vi "T257P_Check_Temperature.vi"(0 "T257P Port IN":refnum<visa-resource-name>, 5 "error in (no error)":errorcluster) -> (7 "Sent buffer 1":string, 11 "Read buffer 1":string, 14 "T257P Port OUT":refnum<visa-resource-name>, 15 "Supply Temperature (C)":dbl format="%.2f", 16 "CheckSum 1":string, 17 "Set Temperature (C)":dbl format="%.2f", 18 "CheckSum 2":string, 19 "error out":errorcluster)   [LabVIEW 2020]
doc: "ThermoTek T257P Labview Driver Library. © G.Shtengel. gleb.shtengel@gmail.com"
panel:
  out "Read buffer 2":string
  out "Loop Counter 2":i32
  out "Sent buffer 2":string
  out "Loop Counter 1":i32
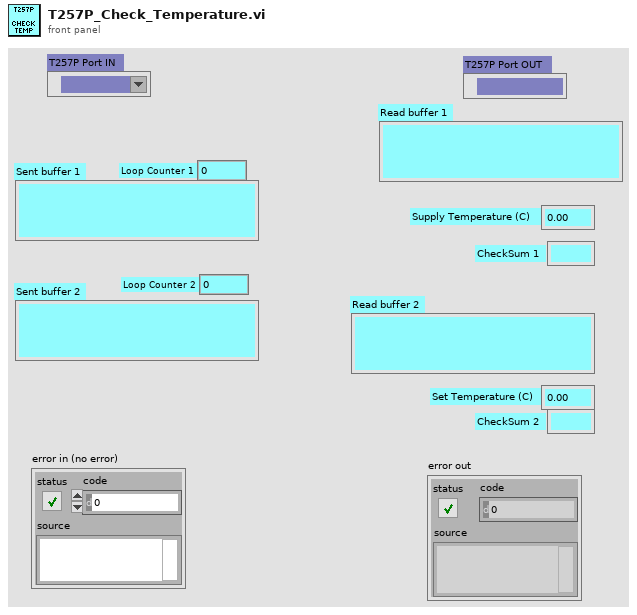
[diagram p1: front panel]
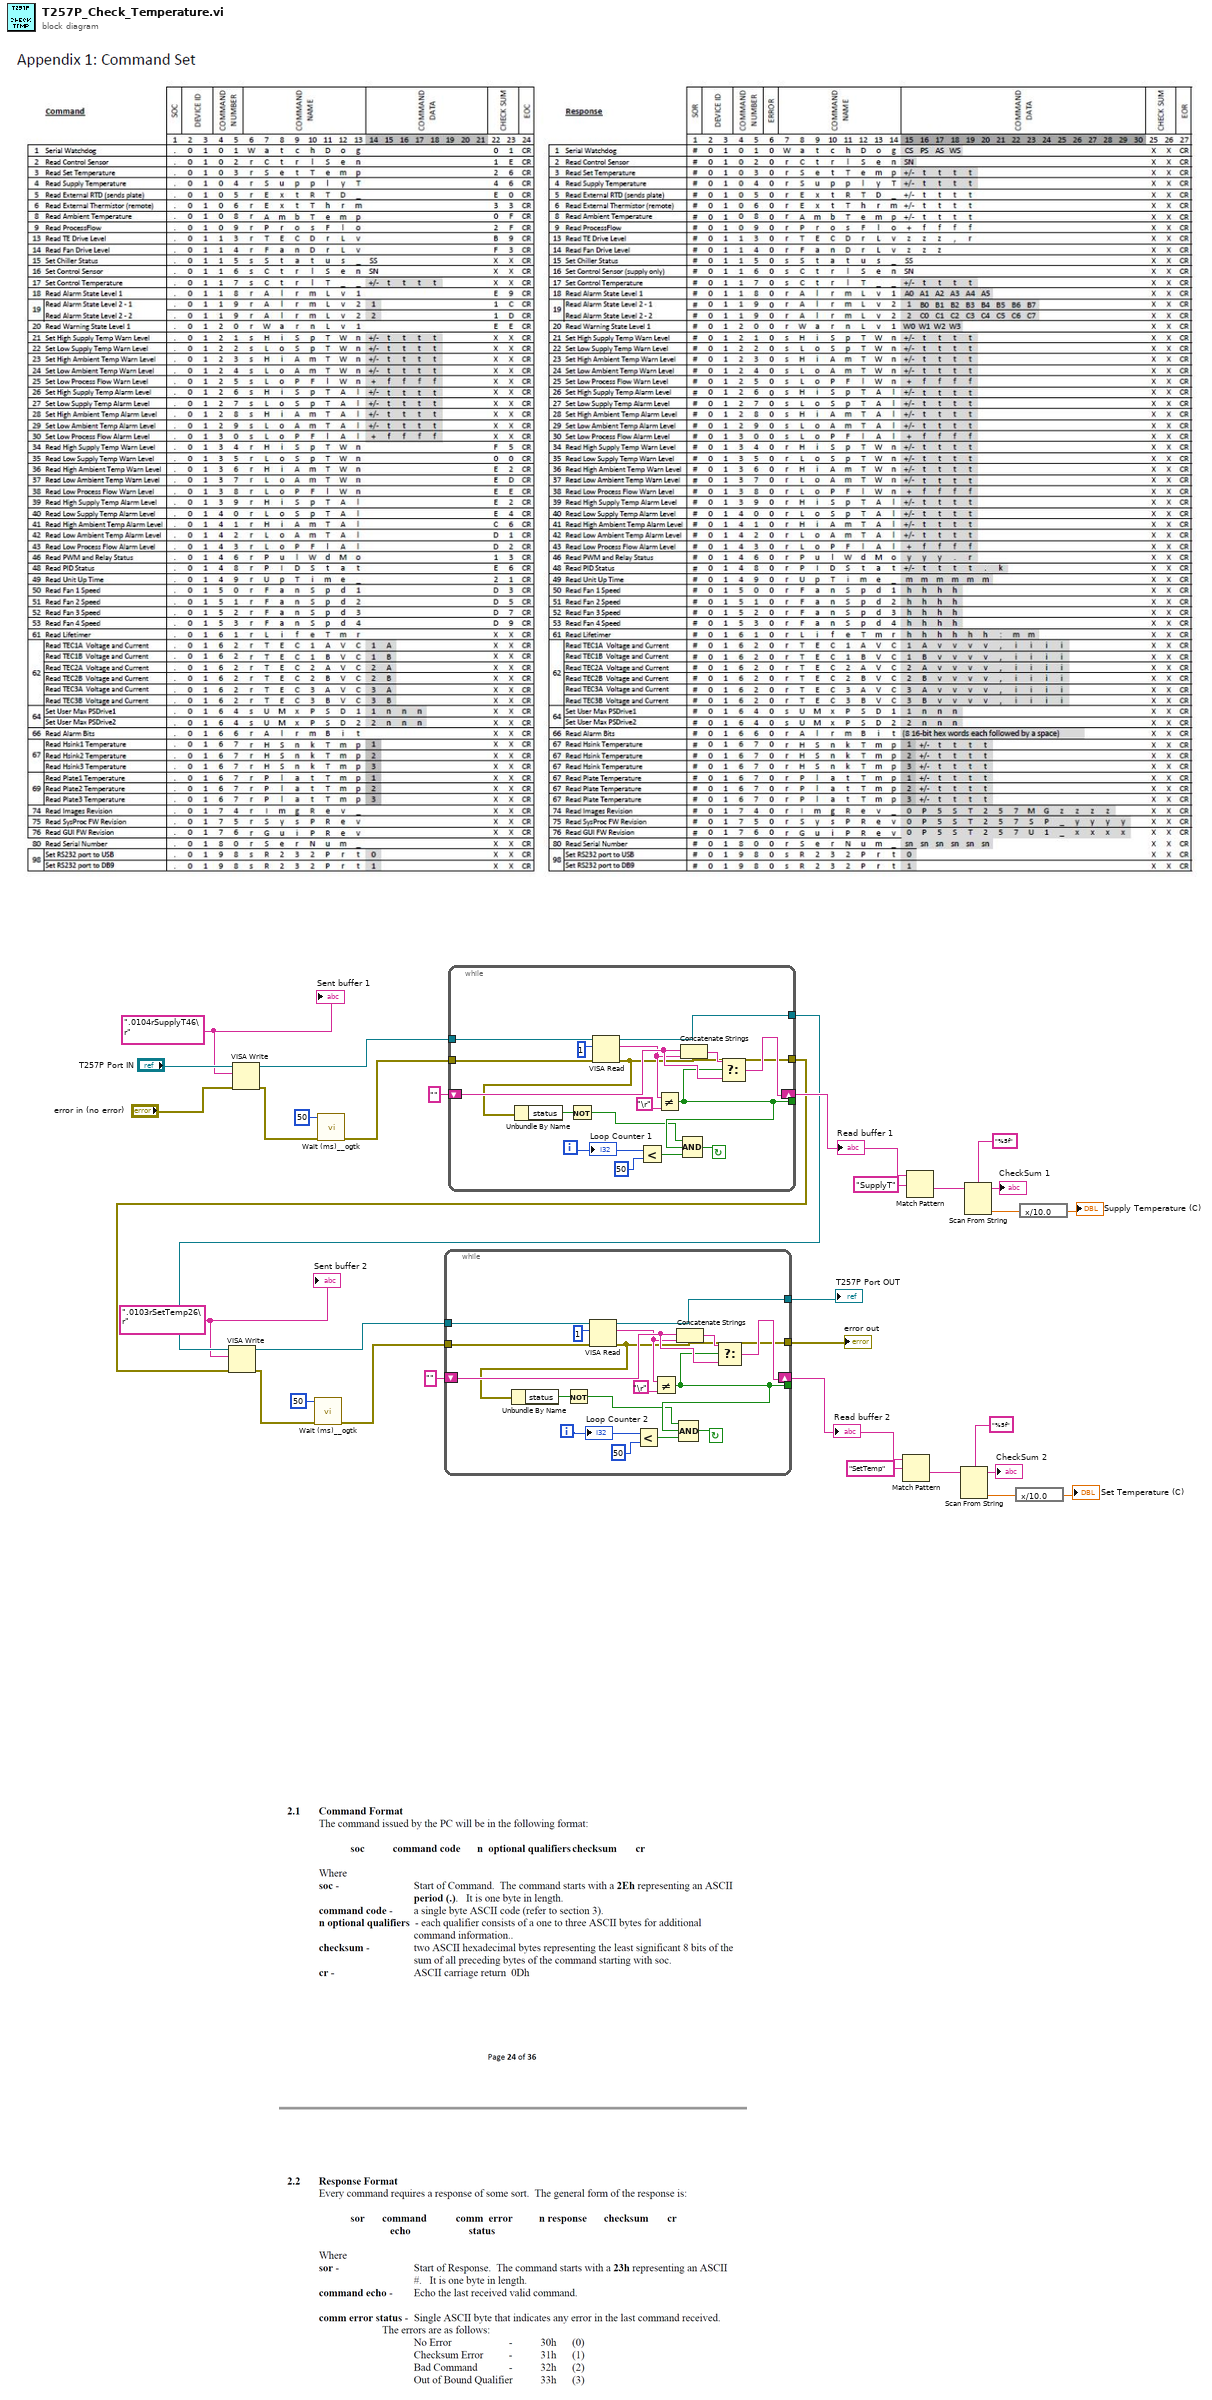
[diagram p0: block diagram]
diagram:
  w1 = ".0103rSetTemp26\r"
  w21 = ".0104rSupplyT46\r"
  n1 = VISA Write(VISA resource name="T257P Port IN", write buffer=w21, error in (no error)="error in (no error)") -> (VISA resource name out=w28:refnum<visa-resource-name>, error out=w29:errorcluster)  [unwired: 1 out]
  n2 = call <userlib>:"Wait (ms)__ogtk.vi"("error in (no error)"=w29, "milliseconds to wait"=u32 50) -> ("error out"=w27:errorcluster)  [unwired: 8 in, 1 out]
  n3 = while {
    shift-left: "" -> [w46]
    shift-right: [w45] -> w22
    tunnel: [w43] -> _
    tunnel: [w35] -> w4
    tunnel: [w44] -> w5
    tunnel: w28 -> [w41]
    tunnel: w27 -> [w40]
    i -> [w42]
    stop <- w47 continue-if-true
    n4 = VISA Read(VISA resource name=w41, byte count=u32 1 ("byte count (0)"), error in (no error)=w40) -> (VISA resource name out=w44:refnum<visa-resource-name>, read buffer=w38:string, error out=w35:errorcluster)  [unwired: 1 out]
    n5 = Unbundle By Name(w35) -> ("status"=w34:bool)
    n6 = Not(x=w34) -> (.not. x?=w33:bool)
    n7 = Less?(x=w42, y=50) -> (x < y?=w48:bool)
    n8 = Not Equal?(x=w38, y="\r") -> (x != y?=w43:bool)
    n9 = Concatenate Strings(w46, w38) -> (w36:string)
    n10 = Compound Arithmetic op=AND(w33, w43, w48) -> (w47:bool)
    n11 = Select(t=w36, s=w43, f=w46) -> (s? t:f=w45:string)
    "Loop Counter 1" <- w42
  }
  "Read buffer 1" <- w22
  n12 = VISA Write(VISA resource name=w5, write buffer=w1, error in (no error)=w4) -> (VISA resource name out=w8:refnum<visa-resource-name>, error out=w7:errorcluster)  [unwired: 1 out]
  n13 = call <userlib>:"Wait (ms)__ogtk.vi"("error in (no error)"=w7, "milliseconds to wait"=u32 50) -> ("error out"=w9:errorcluster)  [unwired: 8 in, 1 out]
  n14 = while {
    shift-left: "" -> [w63]
    shift-right: [w62] -> w14
    tunnel: [w60] -> _
    tunnel: [w52] -> w2
    tunnel: [w61] -> w3
    tunnel: w8 -> [w58]
    tunnel: w9 -> [w57]
    i -> [w59]
    stop <- w64 continue-if-true
    n15 = VISA Read(VISA resource name=w58, byte count=u32 1 ("byte count (0)"), error in (no error)=w57) -> (VISA resource name out=w61:refnum<visa-resource-name>, read buffer=w55:string, error out=w52:errorcluster)  [unwired: 1 out]
    n16 = Unbundle By Name(w52) -> ("status"=w51:bool)
    n17 = Not(x=w51) -> (.not. x?=w50:bool)
    n18 = Less?(x=w59, y=50) -> (x < y?=w65:bool)
    n19 = Not Equal?(x=w55, y="\r") -> (x != y?=w60:bool)
    n20 = Concatenate Strings(w63, w55) -> (w53:string)
    n21 = Compound Arithmetic op=AND(w50, w60, w65) -> (w64:bool)
    n22 = Select(t=w53, s=w60, f=w63) -> (s? t:f=w62:string)
    "Loop Counter 2" <- w59
  }
  "error out" <- w2
  "T257P Port OUT" <- w3
  "Read buffer 2" <- w14
  n23 = Match Pattern(string=w14, regular expression="SetTemp") -> (after substring=w13:string)  [unwired: 1 in, 3 out]
  n24 = Match Pattern(string=w22, regular expression="SupplyT") -> (after substring=w23:string)  [unwired: 1 in, 3 out]
  n25 = Scan From String(format string="%5f", input string=w13) -> (remaining string=→"CheckSum 2":string, output 1=w15:dbl)  [unwired: 3 in, 2 out]
  n26 = Scan From String(format string="%5f", input string=w23) -> (remaining string=→"CheckSum 1":string, output 1=w20:dbl)  [unwired: 3 in, 2 out]
  n27 = expression code="x/10.0"(w15) -> (→"Set Temperature (C)":dbl)
  n28 = expression code="x/10.0"(w20) -> (→"Supply Temperature (C)":dbl)
  "Sent buffer 1" <- w21
  "Sent buffer 2" <- w1
